vi "Configure Stop Trigger [SPT] Core.vi"(7 "Trigger Slope (Positive)":i32(ring) caption="trigger slope (Positive)" items=["Positive", "Negative", "Either"], 8 "error in (no error)":errorcluster, 9 "Trigger Source (None)":string(combo) caption="trigger source (None)", 10 "Channel Name (\"\")":string="CHANNEL1" caption="channel name (\"CHANNEL1\")", 11 "IVI_Fgen in":refnum<class "IVI_Fgen.lvclass">) -> (0 "error out":errorcluster, 3 "IVI_Fgen out":refnum<class "IVI_Fgen.lvclass">)   [LabVIEW 2015, in "IVI_Fgen.lvlib" / "IVI_Fgen.lvclass"]
doc: "This VI configures the properties that control the function generator's stop trigger. These properties are the stop trigger source and slope.\n\nA stop trigger terminates any generation and has the same effect as calling the IviFgen Abort Generation VI.\n\nNote:\n\n(1) This VI is part of the IviFgenStopTrigger [SPT] extension group."
uses:
  IVI_Fgen.lvclass
  IVI_Fgen.lvclass/IVI_Fgen.ctl
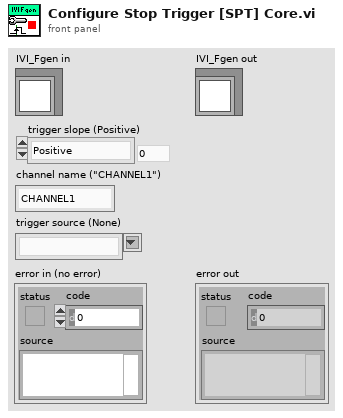
[diagram p1: front panel]
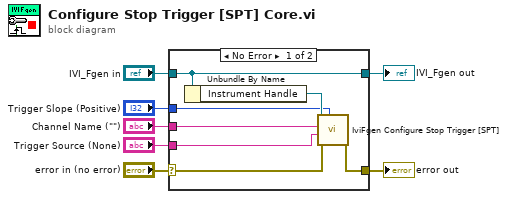
[diagram p0: block diagram]
diagram:
  n1 = case shown="No Error" "error in (no error)" {
    selector: "error in (no error)" -> [w12 w16]
    tunnel: [w11 w16] -> w6
    tunnel: [w14 w15] -> w4
    tunnel: "IVI_Fgen in" -> [w14 w15]
    tunnel: "Trigger Slope (Positive)" -> [w10 _]
    tunnel: "Channel Name (\"\")" -> [w9 _]
    tunnel: "Trigger Source (None)" -> [w8 _]
    frame No Error {
      n2 = Unbundle By Name(w14) -> ("Instrument Handle"=w13:refnum<k15>)
      n3 = call <vilib>:"IviFgen Configure Stop Trigger [SPT].vi"("Trigger Slope (Positive)"=w10, "error in (no error)"=w12, "Trigger Source (None)"=w8, "Channel Name (\"\")"=w9, "instrument handle"=w13) -> ("error out"=w11:errorcluster)  [unwired: 5 in, 1 out]
    }
    frame Error {
    }
  }
  "error out" <- w6
  "IVI_Fgen out" <- w4
